vi "properties.get.vi"(8 "error in (no error)":errorcluster, 11 "Run in":refnum<class "Run.lvclass">) -> (0 "error out":errorcluster, 2 "properties":map{string, string}(c390), 3 "Run out":refnum<class "Run.lvclass">)   [LabVIEW 2020, in "Run.lvclass"]
uses:
  Run.lvclass
  Run.lvclass/Run.ctl
  cd719d9e-4b9a-483f-af8c-e945a04ea9d5.vi
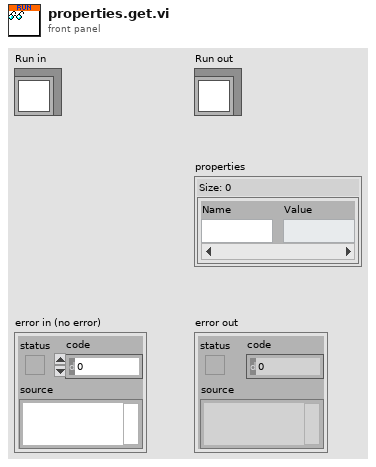
[diagram p1: front panel]
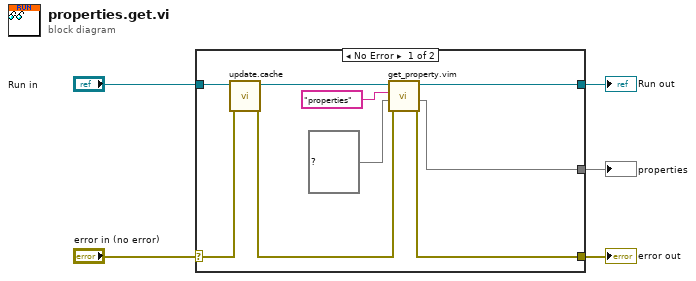
[diagram p0: block diagram]
diagram:
  n1 = case shown="No Error" "error in (no error)" {
    selector: "error in (no error)" -> [w14 w15]
    tunnel: [w9 w15] -> w4
    tunnel: [w8 w16] -> w2
    tunnel: "Run in" -> [w13 w16]
    tunnel: [w6 _] -> w1
    frame No Error {
      n2 = call "update.cache.vi"("error in"=w14, "Run in"=w13) -> ("error out"=w10:errorcluster, "Run out"=w12:refnum<class "Run.lvclass">)  [unwired: 8 in]
      n3 = call "get_property.vim"("error in"=w10, "default value and type"=map{string, string} {} ("properties"), "Property Name"="properties", "Run in"=w12) -> ("error out"=w9:errorcluster, "Value"=w6:map{string, string}, "Run out"=w8:refnum<class "Run.lvclass">)  [unwired: 5 in]
    }
    frame Error {
    }
  }
  "error out" <- w4
  "Run out" <- w2
  "properties" <- w1
